vi "Set State.vi"(8 "error in (no error)":errorcluster, 10 "State":string, 11 "StateMachine in":refnum<class "StateMachine.lvclass">) -> (0 "error out":errorcluster, 3 "StateMachine out":refnum<class "StateMachine.lvclass">)   [LabVIEW 2018, in "State Machine.lvlib" / "StateMachine.lvclass"]
uses:
  StateMachine.lvclass
  StateMachine.lvclass/StateMachine.ctl
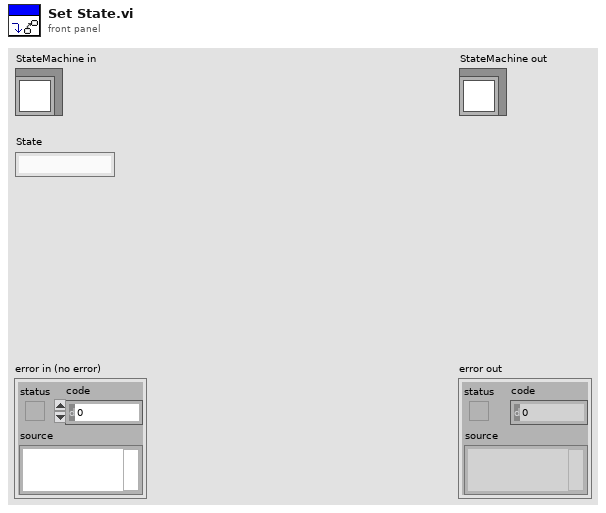
[diagram p1: front panel]
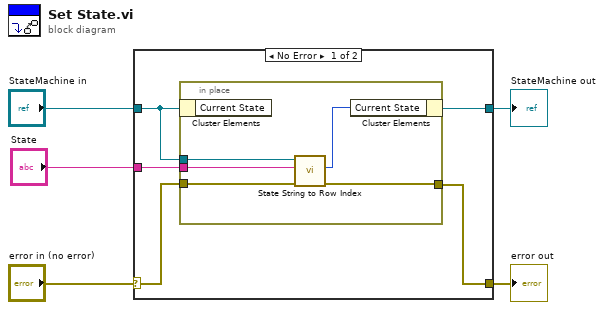
[diagram p0: block diagram]
diagram:
  n1 = case shown="No Error" "error in (no error)" {
    selector: "error in (no error)" -> [w8 w17]
    tunnel: [w7 w17] -> w4
    tunnel: [w6 w16] -> w2
    tunnel: "StateMachine in" -> [w10 w16]
    tunnel: "State" -> [w9 _]
    frame No Error {
      n2 = in-place {
        in-place-border: w10 -> [w14]
        in-place-border: w9 -> [w13]
        in-place-border: w8 -> [w12]
        in-place-border: [w11] -> w7
        n3 = in-place-cluster #1(w10) -> ()  [unwired: 1 out]
        n4 = call-dynamic "State String to Row Index.vi"("error in (no error)"=w12, "State String"=w13, "StateMachine in"=w14) -> ("error out"=w11:errorcluster, "Row Index"=w15:i32)  [unwired: 6 in, 1 out]
        n5 = in-place-cluster #1("Current State"=w15) -> (w6:refnum<class "StateMachine.lvclass">)
      }
    }
    frame Error {
    }
  }
  "error out" <- w4
  "StateMachine out" <- w2
